vi "maxigauge_on_off.vi"(0 "maxi_visa":refnum<visa-resource-name>, 1 "Channel 1":enum16{"NO CHANGE", "OFF", "ON"}(ring), 4 "Channel 2":enum16{"NO CHANGE", "OFF", "ON"}(ring), 5 "err_in":errorcluster, 6 "maxi_delay 2":u32=500, 7 "maxi_delay 3":u32=500, 10 "Channel 3":enum16{"NO CHANGE", "OFF", "ON"}(ring), 11 "Channel 4":enum16{"NO CHANGE", "OFF", "ON"}(ring), 12 "Channel 5":enum16{"NO CHANGE", "OFF", "ON"}(ring), 13 "Channel 6":enum16{"NO CHANGE", "OFF", "ON"}(ring), 18 "maxi_delay":u32=500) -> (14 "GAUGE  Status":string, 19 "err_out":errorcluster)   [LabVIEW 2019]
panel:
  out "Overall Status":bool
  out "Acknowledgement Status":bool
  out "maxi_visa 2":refnum<visa-resource-name>
  in  "maxi_b2r 2":u32
  in  "maxi_b2r":u32
  # "Gauge status:\n1 = OFF\n2 = ON"
  # "VISA"
  # "DELAY"
  # "BYTE AT PORT"
  # "STATUS"
  # "ERROR"
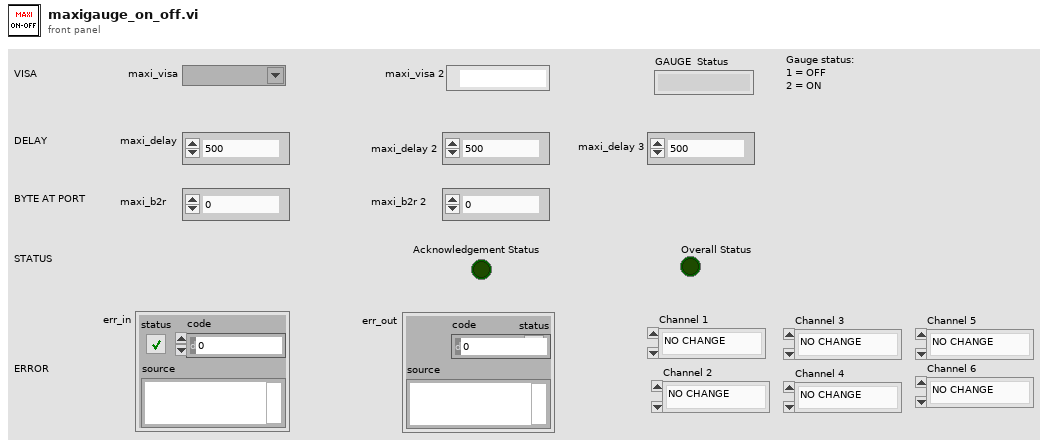
[diagram p1: front panel]
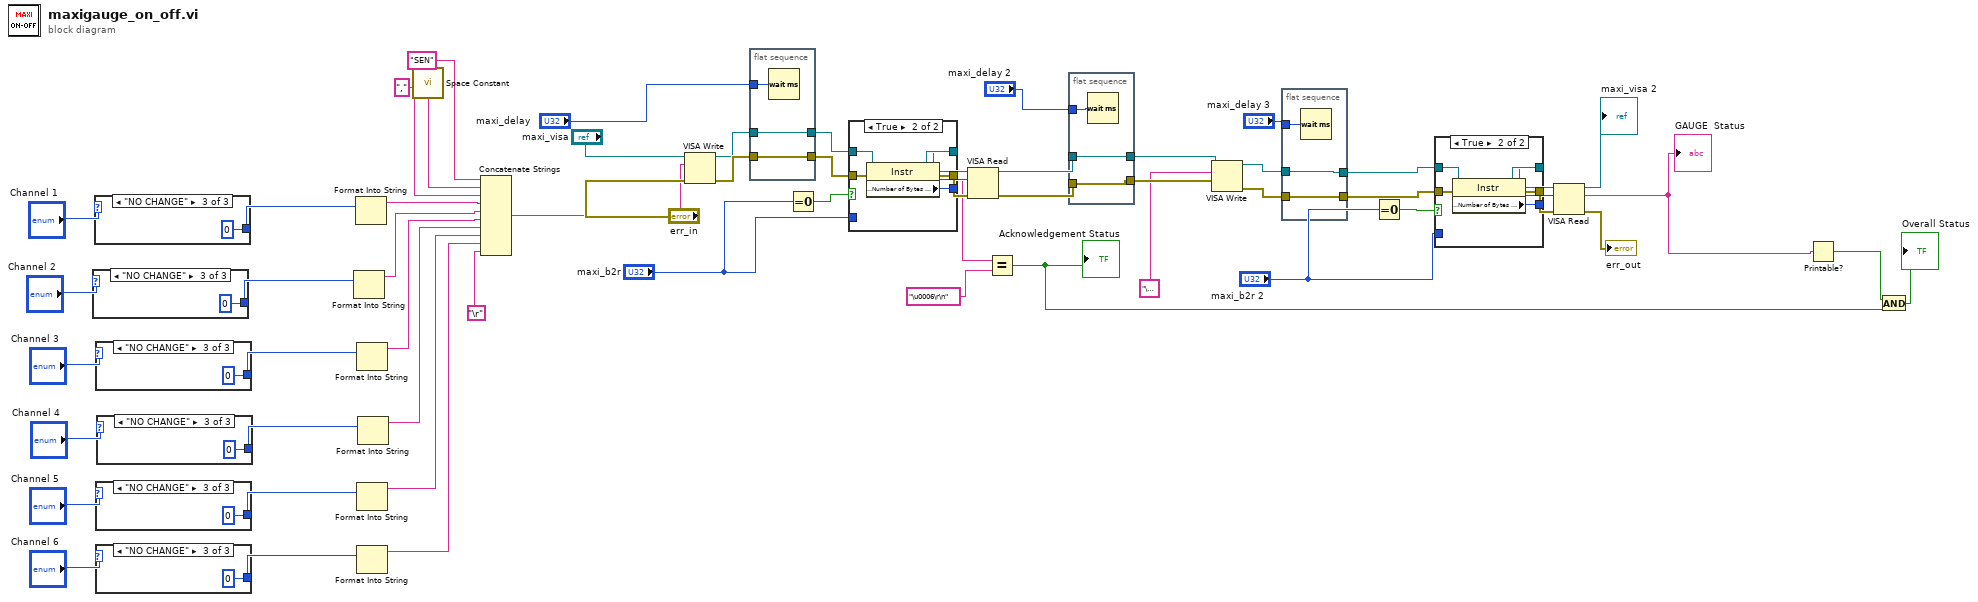
[diagram p0: block diagram]
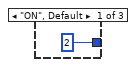
[diagram p2: hidden frame]
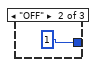
[diagram p3: hidden frame]
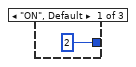
[diagram p4: hidden frame]
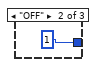
[diagram p5: hidden frame]
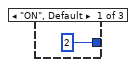
[diagram p6: hidden frame]
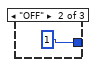
[diagram p7: hidden frame]
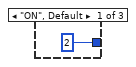
[diagram p8: hidden frame]
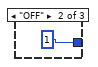
[diagram p9: hidden frame]
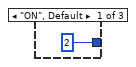
[diagram p10: hidden frame]
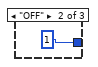
[diagram p11: hidden frame]
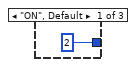
[diagram p12: hidden frame]
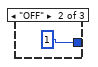
[diagram p13: hidden frame]
diagram:
  n1 = case shown="\"NO CHANGE\"" "Channel 2" {
    tunnel: [2 1 0] -> w14
    frame "ON", Default {
    }
    frame "OFF" {
    }
    frame "NO CHANGE" {
    }
  }
  n2 = case shown="\"NO CHANGE\"" "Channel 1" {
    tunnel: [2 1 0] -> w19
    frame "ON", Default {
    }
    frame "OFF" {
    }
    frame "NO CHANGE" {
    }
  }
  n3 = case shown="\"NO CHANGE\"" "Channel 3" {
    tunnel: [2 1 0] -> w11
    frame "ON", Default {
    }
    frame "OFF" {
    }
    frame "NO CHANGE" {
    }
  }
  n4 = case shown="\"NO CHANGE\"" "Channel 5" {
    tunnel: [2 1 0] -> w5
    frame "ON", Default {
    }
    frame "OFF" {
    }
    frame "NO CHANGE" {
    }
  }
  n5 = case shown="\"NO CHANGE\"" "Channel 6" {
    tunnel: [2 1 0] -> w2
    frame "ON", Default {
    }
    frame "OFF" {
    }
    frame "NO CHANGE" {
    }
  }
  n6 = case shown="\"NO CHANGE\"" "Channel 4" {
    tunnel: [2 1 0] -> w8
    frame "ON", Default {
    }
    frame "OFF" {
    }
    frame "NO CHANGE" {
    }
  }
  n7 = Format Into String(w14) -> (resulting string=w13:string)  [unwired: 3 in, 1 out]
  n8 = Format Into String(w19) -> (resulting string=w17:string)  [unwired: 3 in, 1 out]
  n9 = Format Into String(w11) -> (resulting string=w10:string)  [unwired: 3 in, 1 out]
  n10 = Format Into String(w5) -> (resulting string=w4:string)  [unwired: 3 in, 1 out]
  n11 = Format Into String(w2) -> (resulting string=w1:string)  [unwired: 3 in, 1 out]
  n12 = Format Into String(w8) -> (resulting string=w7:string)  [unwired: 3 in, 1 out]
  n13 = call <vilib>:"Space Constant.vi"() -> ("String"=w20:string)
  n14 = Concatenate Strings("SEN" ("string"), w20, "," ("string"), w17, w13, w10, w7, w4, w1, "\r") -> (w31:string)
  n15 = VISA Write(VISA resource name="maxi_visa", write buffer=w31, error in (no error)="err_in") -> (VISA resource name out=w57:refnum<visa-resource-name>, error out=w59:errorcluster)  [unwired: 1 out]
  n16 = flat-sequence {
    tunnel: w59 -> [w79]
    tunnel: [w79] -> w58
    tunnel: w57 -> [w78]
    tunnel: [w78] -> w56
    tunnel: "maxi_delay" -> [w80]
    frame #0 {
      n17 = Wait (ms)(milliseconds to wait=w80) -> ()  [unwired: 1 out]
    }
  }
  n18 = Equal To 0?(x="maxi_b2r") -> (x = 0?=w52:bool)
  n19 = case shown="True" w52 {
    tunnel: w58 -> [w82 w88]
    tunnel: w56 -> [w83 w87]
    tunnel: [w83 w86] -> w50
    tunnel: [w82 w85] -> w49
    tunnel: [w81 w84] -> w48
    tunnel: "maxi_b2r" -> [w81 _]
    frame False {
    }
    frame True {
      n20 = property class="Instr"(reference=w87, error in=w88) -> (reference out=w86:refnum<visa-resource-name>, error out=w85:errorcluster, "Serial Settings:Number of Bytes at Serial Port"=w84:u32)
    }
  }
  n21 = VISA Read(VISA resource name=w50, byte count=w48, error in (no error)=w49) -> (VISA resource name out=w47:refnum<visa-resource-name>, read buffer=w29:string, error out=w46:errorcluster)  [unwired: 1 out]
  n22 = Equal?(x=w29, y="\u0006\r\n") -> (x = y?=w25:bool)
  "Acknowledgement Status" <- w25
  n23 = flat-sequence {
    tunnel: [w89] -> w44
    tunnel: w47 -> [w91]
    tunnel: [w91] -> w45
    tunnel: "maxi_delay 2" -> [w90]
    tunnel: w46 -> [w89]
    frame #0 {
      n24 = Wait (ms)(milliseconds to wait=w90) -> ()  [unwired: 1 out]
    }
  }
  n25 = VISA Write(VISA resource name=w45, write buffer="\u0005", error in (no error)=w44) -> (VISA resource name out=w37:refnum<visa-resource-name>, error out=w36:errorcluster)  [unwired: 1 out]
  n26 = flat-sequence {
    tunnel: [w93] -> w43
    tunnel: [w94] -> w42
    tunnel: w37 -> [w94]
    tunnel: w36 -> [w93]
    tunnel: "maxi_delay 3" -> [w92]
    frame #0 {
      n27 = Wait (ms)(milliseconds to wait=w92) -> ()  [unwired: 1 out]
    }
  }
  n28 = Equal To 0?(x="maxi_b2r 2") -> (x = 0?=w41:bool)
  n29 = case shown="True" w41 {
    tunnel: w43 -> [w96 w102]
    tunnel: w42 -> [w97 w101]
    tunnel: [w97 w100] -> w40
    tunnel: [w96 w99] -> w39
    tunnel: [w95 w98] -> w38
    tunnel: "maxi_b2r 2" -> [w95 _]
    frame False {
    }
    frame True {
      n30 = property class="Instr"(reference=w101, error in=w102) -> (reference out=w100:refnum<visa-resource-name>, error out=w99:errorcluster, "Serial Settings:Number of Bytes at Serial Port"=w98:u32)
    }
  }
  n31 = VISA Read(VISA resource name=w40, byte count=w38, error in (no error)=w39) -> (VISA resource name out=→"maxi_visa 2":refnum<visa-resource-name>, read buffer=w23:string, error out=→"err_out":errorcluster)  [unwired: 1 out]
  "GAUGE  Status" <- w23
  n32 = Printable?(1:w23) -> (0:w22:bool)
  n33 = And(x=w22, y=w25) -> (x .and. y?=→"Overall Status":bool)
